vi "Encoders.vi"(1 "Number of Encoders":i32=1 min=1 max=5, 2 "Reset":bool, 3 "Inversions":bool[](array[boolean])=[FALSE], 4 "Mode":enum8{"Start", "Run", "Finish"}(ring)) -> (0 "Encoder":T1(array[cluster]))   [LabVIEW 2014]
uses:
  <vilib>/Rock Robotics/WPI/Counter/WPI_CounterDigitalInputToDigitalSource.vi
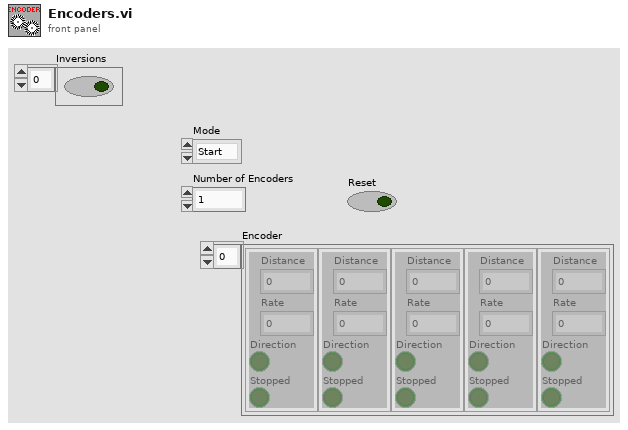
[diagram p1: front panel]
types:
  T1 = cluster{"Distance":dbl, "Rate":dbl, "Direction":bool, "Stopped":bool}[]
  T2 = cluster{"Distance":dbl, "Rate":dbl, "Direction":bool, "Stopped":bool}
  T3 = typedef "WPI_EncoderDevRef.ctl" = cluster{"DevStatus":errorcluster, "EncoderIndex":T4, "CounterIndex":T5, "DistancePerCount":dbl, "Decoding Type":T6}
  T4 = typedef "FPGA_EncoderIdx.ctl" = enum8{"Enc 0", "Enc 1", "Enc 2", "Enc 3", "Enc 4", "Enc 5", "Enc 6", "Enc 7", "Invalid"}
  T5 = typedef "FPGA_CounterCtrSystemIndex.ctl" = enum8{"Ctr 0", "Ctr 1", "Ctr 2", "Ctr 3", "Ctr 4", "Ctr 5", "Ctr 6", "Ctr 7", "Invalid"}
  T6 = typedef "WPI_EncoderType.ctl" = enum16{"1x", "2x", "4x"}
  T7 = typedef "WPI_DigitalInputDevRef.ctl" = cluster{"DevStatus":errorcluster, "DIO Channel":T8, "Controller":T9}
  T8 = typedef "FPGA_DIOChannel.ctl" = enum8{"DIO 0", "DIO 1", "DIO 2", "DIO 3", "DIO 4", "DIO 5", "DIO 6", "DIO 7", "DIO 8", "DIO 9", "DIO MXP 0", "DIO MXP 1", "DIO MXP 2", "DIO MXP 3", "DIO MXP 4", "DIO MXP 5", "DIO MXP 6", "DIO MXP 7", "DIO MXP 8", "DIO MXP 9", "DIO MXP 10", "DIO MXP 11", "DIO MXP 12", "DIO MXP 13", "DIO MXP 14", "DIO MXP 15", "Invalid"}
  T9 = typedef "FPGA_TypedefDigitalModule.ctl" = enum16{"Controller 1"}
  T10 = typedef "FPGA_CounterEncoderSourceConvertionLVSourceType.ctl" = cluster{"DevStatus":errorcluster, "AnalogTriggerMode?":bool, "DigitalMode":cluster{"Controller":T9, "DIO Channel":T11}, "AnalogTriggerMode":cluster{"AnalogTriggerIndex":T12, "OutputType":T13}}
  T11 = typedef "FPGA_DIODigitalSourceChannel.ctl" = enum8{"DIO 0", "DIO 1", "DIO 2", "DIO 3", "DIO 4", "DIO 5", "DIO 6", "DIO 7", "DIO 8", "DIO 9", "DIO MXP 0", "DIO MXP 1", "DIO MXP 2", "DIO MXP 3", "DIO MXP 4", "DIO MXP 5", "DIO MXP 6", "DIO MXP 7", "DIO MXP 8", "DIO MXP 9", "DIO MXP 10", "DIO MXP 11", "DIO MXP 12", "DIO MXP 13", "DIO MXP 14", "DIO MXP 15", "Disabled"}
  T12 = typedef "FPGA_AnalogTriggerIndex.ctl" = enum8{"Trig 0", "Trig 1", "Trig 2", "Trig 3", "Trig 4", "Trig 5", "Trig 6", "Trig 7", "Invalid"}
  T13 = typedef "FPGA_AnalogTriggerOutType.ctl" = enum16{"InWindow", "TriggerState", "Rising", "Falling"}
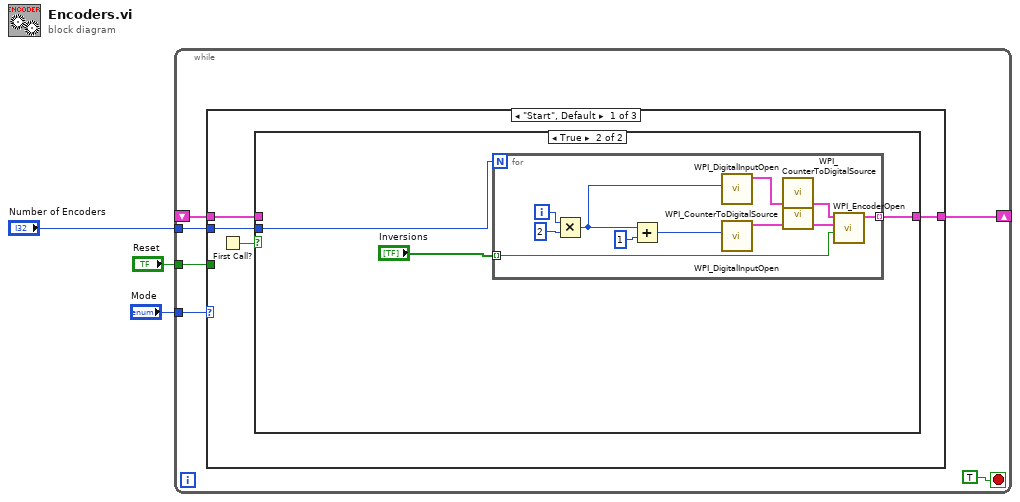
[diagram p0: block diagram]
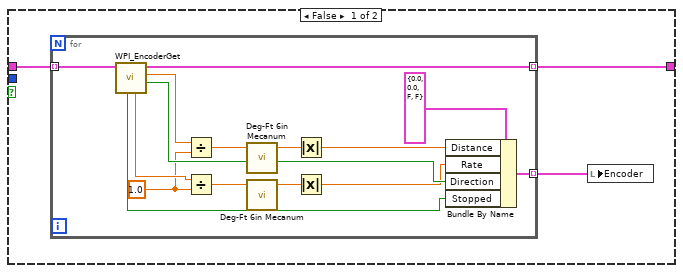
[diagram p2: hidden frame]
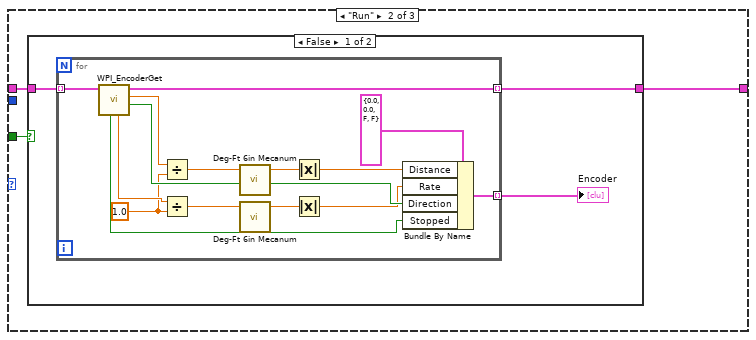
[diagram p3: hidden frame]
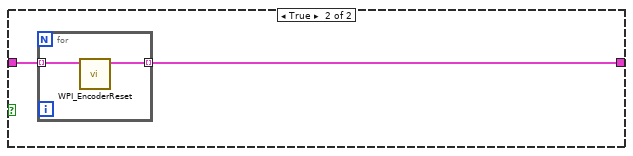
[diagram p4: hidden frame]
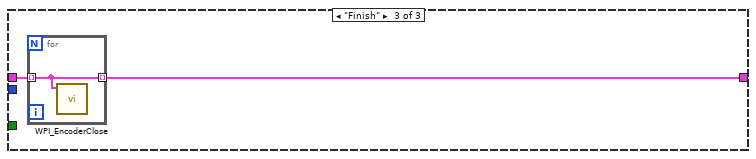
[diagram p5: hidden frame]
diagram:
  n1 = while {
    tunnel: "Number of Encoders" -> [w9]
    tunnel: "Mode" -> [w8]
    shift-right: [w7] -> _
    shift-left: _ -> [w6]
    tunnel: "Reset" -> [w4]
    stop <- TRUE stop-if-true
    n2 = case shown="\"Start\", Default" w8 {
      tunnel: w9 -> [w13 _ _]
      tunnel: [w12 w47 w71] -> w7
      tunnel: w6 -> [w10 w48 w72]
      tunnel: w4 -> [_ w46 _]
      frame "Start", Default {
        n3 = First Call?() -> (First Call?: T/F=w11:bool)
        n4 = case shown="True" w11 {
          tunnel: w13 -> [_ w34]
          tunnel: [w15 w33] -> w12
          tunnel: w10 -> [w16 _]
          frame False {
            n5 = for {
              tunnel: w16 -> [w31] mode=indexing
              tunnel: [w30] -> w15 mode=indexing
              tunnel: [w26] -> w14 mode=indexing
              w23 = 1.0 ("y")
              n6 = call <vilib>:"WPI_EncoderGet.vi"("EncoderDevRef"=w31) -> ("Direction"=w28:bool, "Distance"=w25:dbl, "EncoderDevRef"=w30:T3, "Rate"=w24:dbl, "Stopped"=w27:bool)  [unwired: 5 in, 1 out]
              n7 = Divide(x=w25, y=w23) -> (x/y=w21:dbl)
              n8 = Divide(x=w24, y=w23) -> (x/y=w22:dbl)
              n9 = call "Deg-Ft 6in Mecanum.vi"("Input"=w21) -> ("Output"=w20:dbl)  [unwired: 4 in]
              n10 = call "Deg-Ft 6in Mecanum.vi"("Input"=w22) -> ("Output"=w19:dbl)  [unwired: 4 in]
              n11 = Absolute Value(x=w20) -> (abs(x)=w18:dbl)
              n12 = Absolute Value(x=w19) -> (abs(x)=w17:dbl)
              n13 = Bundle By Name(cluster=T2 {"Distance"=0.0, "Rate"=0.0, "Direction"=FALSE, "Stopped"=FALSE} ("Encoder"), "Distance"=w18, "Rate"=w17, "Direction"=w28, "Stopped"=w27) -> (w26:T2)
            }
            n14 = local write "Encoder"(w14) -> ()
          }
          frame True {
            n15 = for {
              N: w34 -> [_]
              tunnel: [w36] -> w33 mode=indexing
              tunnel: "Inversions" -> [w35] mode=indexing
              i -> [w41]
              n16 = Multiply(x=w41, y=2) -> (x*y=w38:i32)
              n17 = Add(x=w38, y=1) -> (x+y=w39:i32)
              n18 = call <vilib>:"WPI_DigitalInputOpen.vi"("DIO Channel"=w38) -> ("DigitalInputDevRef"=w43:T7)  [unwired: 2 in, 8 out]
              n19 = call <vilib>:"WPI_DigitalInputOpen.vi"("DIO Channel"=w39) -> ("DigitalInputDevRef"=w44:T7)  [unwired: 2 in, 8 out]
              n20 = call-poly <vilib>:"WPI_CounterToDigitalSource.vi"("DigitalInputDevRef"=w43) -> ("Digital Source"=w42:T10)  [unwired: 6 out]
              n21 = call-poly <vilib>:"WPI_CounterToDigitalSource.vi"("DigitalInputDevRef"=w44) -> ("Digital Source"=w45:T10)  [unwired: 6 out]
              n22 = call <vilib>:"WPI_EncoderOpen.vi"("Invert Direction (False)"=w35, "BSource"=w45, "ASource"=w42) -> ("EncoderDevRef"=w36:T3)  [unwired: 5 in, 3 out]
            }
          }
        }
      }
      frame "Run" {
        n23 = case shown="False" w46 {
          tunnel: w48 -> [w51 w68]
          tunnel: [w50 w67] -> w47
          frame False {
            n24 = for {
              tunnel: w51 -> [w66] mode=indexing
              tunnel: [w65] -> w50 mode=indexing
              tunnel: [w61] -> w49 mode=indexing
              w58 = 1.0 ("y")
              n25 = call <vilib>:"WPI_EncoderGet.vi"("EncoderDevRef"=w66) -> ("Direction"=w63:bool, "Distance"=w60:dbl, "EncoderDevRef"=w65:T3, "Rate"=w59:dbl, "Stopped"=w62:bool)  [unwired: 5 in, 1 out]
              n26 = Divide(x=w60, y=w58) -> (x/y=w56:dbl)
              n27 = Divide(x=w59, y=w58) -> (x/y=w57:dbl)
              n28 = call "Deg-Ft 6in Mecanum.vi"("Input"=w56) -> ("Output"=w55:dbl)  [unwired: 4 in]
              n29 = call "Deg-Ft 6in Mecanum.vi"("Input"=w57) -> ("Output"=w54:dbl)  [unwired: 4 in]
              n30 = Absolute Value(x=w55) -> (abs(x)=w53:dbl)
              n31 = Absolute Value(x=w54) -> (abs(x)=w52:dbl)
              n32 = Bundle By Name(cluster=T2 {"Distance"=0.0, "Rate"=0.0, "Direction"=FALSE, "Stopped"=FALSE} ("Encoder"), "Distance"=w53, "Rate"=w52, "Direction"=w63, "Stopped"=w62) -> (w61:T2)
            }
            "Encoder" <- w49
          }
          frame True {
            n33 = for {
              tunnel: [w69] -> w67 mode=indexing
              tunnel: w68 -> [w70] mode=indexing
              n34 = call <vilib>:"WPI_EncoderReset.vi"("EncoderDevRef"=w70) -> ("EncoderDevRef"=w69:T3)  [unwired: 9 in, 1 out]
            }
          }
        }
      }
      frame "Finish" {
        n35 = for {
          tunnel: [w73] -> w71 mode=indexing
          tunnel: w72 -> [w73] mode=indexing
          n36 = call <vilib>:"WPI_EncoderClose.vi"("EncoderDevRef"=w73) -> ()  [unwired: 10 in, 1 out]
        }
      }
    }
  }
